vi "substitution.vi"(4 "polynomial equation 2":T1, 5 "polynomial equation 1":T1) -> (0 "successful?":bool, 1 "polynomial equation 1":T1)   [LabVIEW 2009]
uses:
  polynomial equation.ctl
panel:
  # "substitues eqation 2 into equation 1"
  # "currently trims arrays to smallest size"
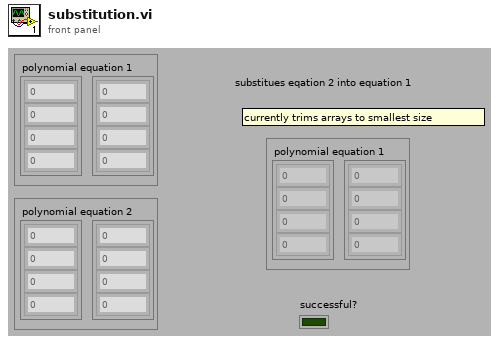
[diagram p1: front panel]
types:
  T1 = typedef "polynomial equation.ctl" = cluster{"i":dbl[], "ii":dbl[]}
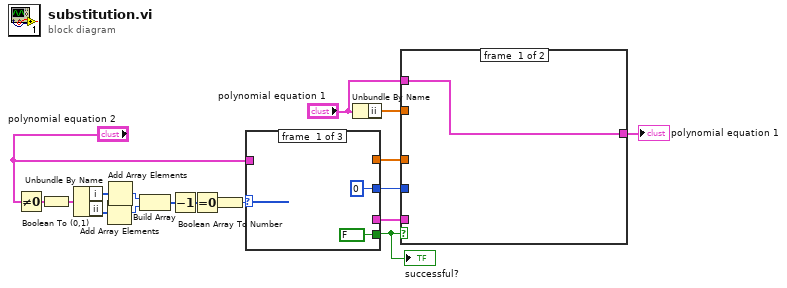
[diagram p0: block diagram]
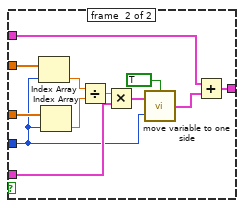
[diagram p2: hidden frame]
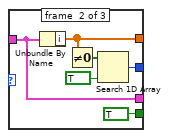
[diagram p3: hidden frame]
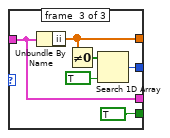
[diagram p4: hidden frame]
diagram:
  n1 = Not Equal To 0?(x="polynomial equation 2") -> (x != 0?=w13:cluster{"i":bool[], "ii":bool[]})
  n2 = Boolean To (0,1)(Boolean=w13) -> (0, 1=w12:cluster{"i":i16[], "ii":i16[]})
  n3 = Unbundle By Name(w12) -> ("i"=w11:i16[], "ii"=w10:i16[])
  n4 = Add Array Elements(numeric array=w10) -> (sum=w7:i16)
  n5 = Add Array Elements(numeric array=w11) -> (sum=w8:i16)
  n6 = Build Array(w8, w7) -> (w6:i16[])
  n7 = Decrement(x=w6) -> (x-1=w9:i16[])
  n8 = Equal To 0?(x=w9) -> (x = 0?=w5:bool[])
  n9 = Boolean Array To Number(Boolean array=w5) -> (number=w2:u32)
  n10 = case shown="2" w2 {
    tunnel: [_ w23 w29] -> w18
    tunnel: [0 ("index") w24 w30] -> w16
    tunnel: "polynomial equation 2" -> [_ w26 w32]
    tunnel: [_ w26 w32] -> w3
    tunnel: [FALSE TRUE TRUE] -> w1
    frame #0 {
    }
    frame #1 {
      n11 = Unbundle By Name(w26) -> ("i"=w23:dbl[])
      n12 = Not Equal To 0?(x=w23) -> (x != 0?=w22:bool[])
      n13 = Search 1D Array(1D array=w22, element=TRUE) -> (index of element=w24:i32)  [unwired: 1 in]
    }
    frame #2 {
      n14 = Unbundle By Name(w32) -> ("ii"=w29:dbl[])
      n15 = Not Equal To 0?(x=w29) -> (x != 0?=w28:bool[])
      n16 = Search 1D Array(1D array=w28, element=TRUE) -> (index of element=w30:i32)  [unwired: 1 in]
    }
  }
  "successful?" <- w1
  n17 = Unbundle By Name("polynomial equation 1") -> ("ii"=w17:dbl[])
  n18 = case shown="True" w1 {
    tunnel: w18 -> [_ w45]
    tunnel: w17 -> [_ w44]
    tunnel: w16 -> [_ w34]
    tunnel: "polynomial equation 1" -> [w33 w37]
    tunnel: [w33 w36] -> w14
    tunnel: w3 -> [_ w35]
    frame #0 {
    }
    frame #1 {
      n19 = Index Array(array=w44, index=w34) -> (element=w42:dbl)
      n20 = Index Array(array=w45, index=w34) -> (element=w43:dbl)
      n21 = Divide(x=w42, y=w43) -> (x/y=w41:dbl)
      n22 = Multiply(x=w41, y=w35) -> (x*y=w40:T1)
      n23 = call "move variable to one side.vi"("i to ii ? (ii to i)"=TRUE, "index"=w34, "system of equation"=w40) -> ("system of equation"=w38:T1)
      n24 = Add(x=w37, y=w38) -> (x+y=w36:T1)
    }
  }
  "polynomial equation 1" <- w14
